vi "Include_Defocus_for_SphAb_v1.vi"(1 "amplitude in":dbl[](array[numeric])) -> (0 "amplitude out":dbl[](array[numeric]))   [LabVIEW 2015]
panel:
  in  "Defocus relative to 2nd Order SphAb":dbl format="%#_13g"
  in  "Defocus relative to 1st Order SphAb":dbl format="%#_13g"
  in  "Ratio of SphAb 2nd / 1st":dbl format="%#_13g"
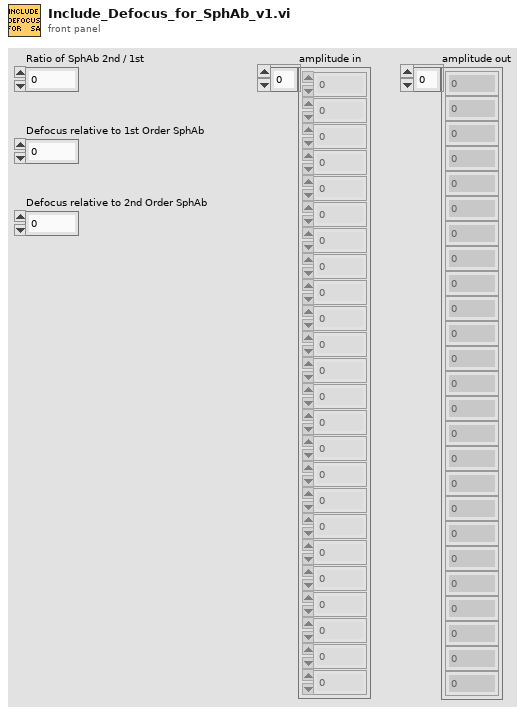
[diagram p1: front panel]
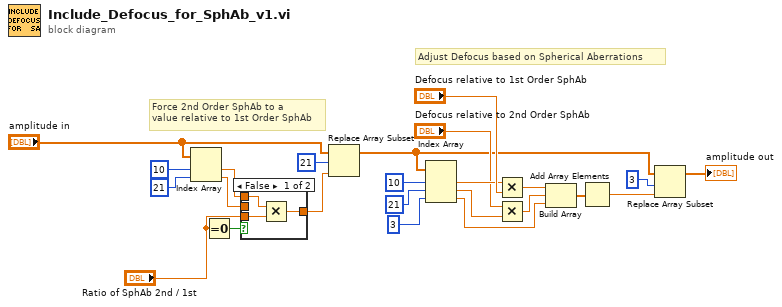
[diagram p0: block diagram]
diagram:
  # "Force 2nd Order SphAb to a \nvalue relative to 1st Order SphAb"
  # "Adjust Defocus based on Spherical Aberrations"
  n1 = Index Array(array="amplitude in", index #1=10 ("index"), index #2=21 ("index")) -> (element #1=w4:dbl, element #2=w1:dbl)
  n2 = Equal To 0?(x="Ratio of SphAb 2nd / 1st") -> (x = 0?=w6:bool)
  n3 = case shown="False" w6 {
    tunnel: "Ratio of SphAb 2nd / 1st" -> [w27 _]
    tunnel: w4 -> [w26 _]
    tunnel: [w25 w28] -> w3
    tunnel: w1 -> [_ w28]
    frame False {
      n4 = Multiply(x=w26, y=w27) -> (x*y=w25:dbl)
    }
    frame True {
    }
  }
  n5 = Replace Array Subset(array="amplitude in", new element=w3, index=21) -> (w7:dbl[])
  n6 = Index Array(array=w7, index #1=10 ("index"), index #2=21 ("index"), index #3=3 ("index")) -> (element #1=w21:dbl, element #2=w17:dbl, element #3=w12:dbl)
  n7 = Multiply(x=w21, y="Defocus relative to 1st Order SphAb") -> (x*y=w14:dbl)
  n8 = Multiply(x="Defocus relative to 2nd Order SphAb", y=w17) -> (x*y=w13:dbl)
  n9 = Build Array(w14, w13, w12) -> (w15:dbl[])
  n10 = Add Array Elements(numeric array=w15) -> (sum=w11:dbl)
  n11 = Replace Array Subset(array=w7, new element=w11, index=3) -> (→"amplitude out":dbl[])
